vi "fits_header.vi"(0 "gfits refnum":T1, 2 "wavelength":dbl=630.2, 3 "Instru ID":string="MSSP_FeI", 4 "error in (no error)":errorcluster, 5 "start time":timestamp, 6 "total scans":dbl=190.0, 7 "end time":timestamp, 8 "Exposure":i32, 9 "num of img added":i32=1, 10 "lcvr1_2":dbl, 11 "lcvr2_4":dbl, 12 "lcvr1_4":dbl, 13 "lcvr2_2":dbl, 14 "lcvr1_1":dbl, 15 "lcvr1_3":dbl, 16 "lcvr2_1":dbl, 17 "lcvr2_3":dbl, 18 "Curr Scan":dbl, 19 "Teliscope parameters":bool) -> (20 "dup gfits refnum":T1, 27 "error out":errorcluster)   [LabVIEW 2014]
uses:
  gfitsio/gfitsio-refnum.ctl
  gfitsio/gfitsio.lvlib
  weekend/mast_controlsystem/MASTTCSGET.lvlib
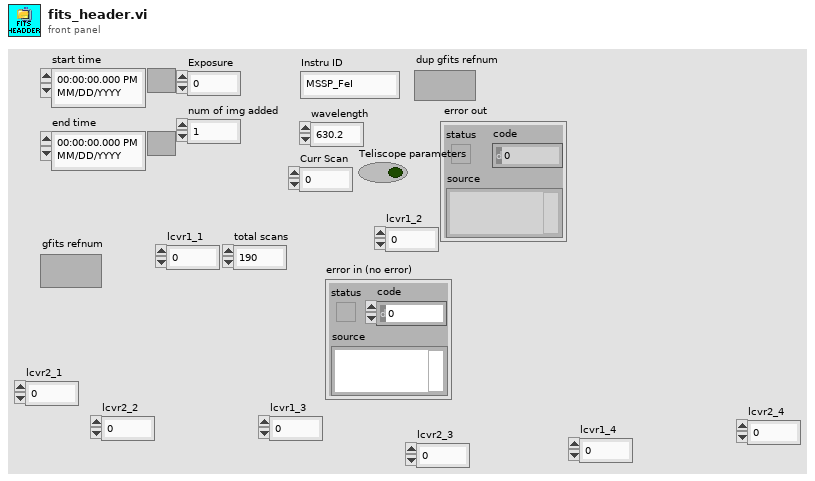
[diagram p1: front panel]
types:
  T1 = typedef "gfitsio.lvlib/gfitsio-refnum.ctl" = refnum<k1>
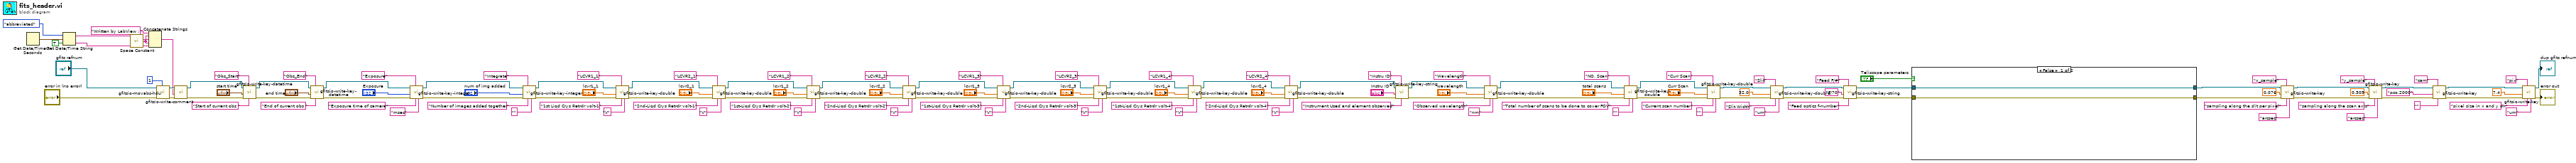
[diagram p0: block diagram]
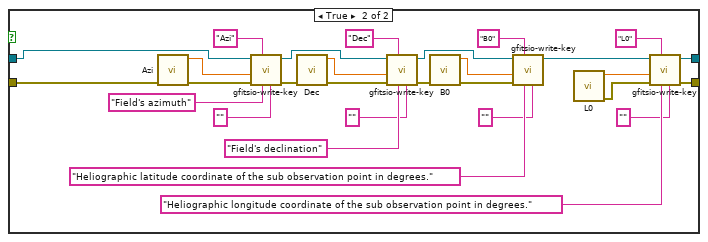
[diagram p2: hidden frame]
diagram:
  n1 = Get Date/Time In Seconds() -> (seconds since 1Jan1904=w143:timestamp)
  n2 = Get Date/Time String(date format (0)=enum16{"short", "long", "abbreviated"}."abbreviated", seconds (now)=w143, want seconds? (F)=TRUE) -> (date string=w140:string, time string=w138:string)
  n3 = call <vilib>:"Space Constant.vi"() -> ("String"=w139:string)
  n4 = Concatenate Strings("Written by LabView : " ("comment"), w139, w140, w139, w138) -> (w136:string)
  n5 = call "gfitsio-movabs-hdu.vi"("hdunum"=1, "error in (no error)"="error in (no error)", "gfits refnum"="gfits refnum") -> ("error out"=w135:errorcluster, "dup gfits refnum"=w137:T1)  [unwired: 6 in, 1 out]
  n6 = call "gfitsio-write-comment.vi"("error in (no error)"=w135, "comment"=w136, "gfits refnum"=w137) -> ("error out"=w131:errorcluster, "dup gfits refnum"=w132:T1)  [unwired: 7 in]
  n7 = call "gfitsio-write-key-datetime.vi"("comment"="Start of current obs ", "keyname"="Obs_Start", "error in (no error)"=w131, "value"="start time", "gfits refnum"=w132) -> ("error out"=w127:errorcluster, "dup gfits refnum"=w130:T1)  [unwired: 5 in]
  n8 = call "gfitsio-write-key-datetime.vi"("comment"="End of current obs ", "keyname"="Obs_End", "error in (no error)"=w127, "value"="end time", "gfits refnum"=w130) -> ("error out"=w125:errorcluster, "dup gfits refnum"=w126:T1)  [unwired: 5 in]
  n9 = call "gfitsio-write-key-integer.vi"("units"="msec", "comment"="Exposure time of camera", "keyname"="Exposure", "error in (no error)"=w125, "value"="Exposure", "gfits refnum"=w126) -> ("error out"=w114:errorcluster, "dup gfits refnum"=w118:T1)  [unwired: 4 in]
  n10 = call "gfitsio-write-key-integer.vi"("units"="", "comment"="Number of images added together", "keyname"="Integrate", "error in (no error)"=w114, "value"="num of img added", "gfits refnum"=w118) -> ("error out"=w112:errorcluster, "dup gfits refnum"=w113:T1)  [unwired: 4 in]
  n11 = call "gfitsio-write-key-double.vi"("units"="V", "comment"="1st Liqd Crys Retrdr volt-1", "keyname"="LCVR1_1", "error in (no error)"=w112, "value"="lcvr1_1", "gfits refnum"=w113) -> ("error out"=w102:errorcluster, "dup gfits refnum"=w103:T1)  [unwired: 4 in]
  n12 = call "gfitsio-write-key-double.vi"("units"="V", "comment"="2nd-Liqd Crys Retrdr volt-1", "keyname"="LCVR2_1", "error in (no error)"=w102, "value"="lcvr2_1", "gfits refnum"=w103) -> ("error out"=w96:errorcluster, "dup gfits refnum"=w97:T1)  [unwired: 4 in]
  n13 = call "gfitsio-write-key-double.vi"("units"="V", "comment"="1st-Liqd Crys Retrdr volt-2", "keyname"="LCVR1_2", "error in (no error)"=w96, "value"="lcvr1_2", "gfits refnum"=w97) -> ("error out"=w74:errorcluster, "dup gfits refnum"=w75:T1)  [unwired: 4 in]
  n14 = call "gfitsio-write-key-double.vi"("units"="V", "comment"="2nd-Liqd Crys Retrdr volt-2", "keyname"="LCVR2_2", "error in (no error)"=w74, "value"="lcvr2_2", "gfits refnum"=w75) -> ("error out"=w72:errorcluster, "dup gfits refnum"=w73:T1)  [unwired: 4 in]
  n15 = call "gfitsio-write-key-double.vi"("units"="V", "comment"="1st-Liqd Crys Retrdr volt-3", "keyname"="LCVR1_3", "error in (no error)"=w72, "value"="lcvr1_3", "gfits refnum"=w73) -> ("error out"=w70:errorcluster, "dup gfits refnum"=w71:T1)  [unwired: 4 in]
  n16 = call "gfitsio-write-key-double.vi"("units"="V", "comment"="2nd-Liqd Crys Retrdr volt-3", "keyname"="LCVR2_3", "error in (no error)"=w70, "value"="lcvr2_3", "gfits refnum"=w71) -> ("error out"=w68:errorcluster, "dup gfits refnum"=w69:T1)  [unwired: 4 in]
  n17 = call "gfitsio-write-key-double.vi"("units"="V", "comment"="1st-Liqd Crys Retrdr volt-4", "keyname"="LCVR1_4", "error in (no error)"=w68, "value"="lcvr1_4", "gfits refnum"=w69) -> ("error out"=w66:errorcluster, "dup gfits refnum"=w67:T1)  [unwired: 4 in]
  n18 = call "gfitsio-write-key-double.vi"("units"="V", "comment"="2nd-Liqd Crys Retrdr volt-4", "keyname"="LCVR2_4", "error in (no error)"=w66, "value"="lcvr2_4", "gfits refnum"=w67) -> ("error out"=w61:errorcluster, "dup gfits refnum"=w62:T1)  [unwired: 4 in]
  n19 = call "gfitsio-write-key-string.vi"("comment"="Instrument Used and element observed", "keyname"="Instru ID", "error in (no error)"=w61, "value"="Instru ID", "gfits refnum"=w62) -> ("error out"=w59:errorcluster, "dup gfits refnum"=w60:T1)  [unwired: 5 in]
  n20 = call "gfitsio-write-key-double.vi"("units"="nm", "comment"="Observed wavelength", "keyname"="Wavelength", "error in (no error)"=w59, "value"="wavelength", "gfits refnum"=w60) -> ("error out"=w51:errorcluster, "dup gfits refnum"=w54:T1)  [unwired: 4 in]
  n21 = call "gfitsio-write-key-double.vi"("units"="", "comment"="Total number of scans to be done to cover FOV", "keyname"="NO. Scan", "error in (no error)"=w51, "value"="total scans", "gfits refnum"=w54) -> ("error out"=w46:errorcluster, "dup gfits refnum"=w47:T1)  [unwired: 4 in]
  n22 = call "gfitsio-write-key-double.vi"("units"="", "comment"="Current scan number", "keyname"="Curr Scan", "error in (no error)"=w46, "value"="Curr Scan", "gfits refnum"=w47) -> ("error out"=w40:errorcluster, "dup gfits refnum"=w43:T1)  [unwired: 4 in]
  n23 = call "gfitsio-write-key-double.vi"("units"="um", "comment"="Slit Width", "keyname"="Slit", "error in (no error)"=w40, "value"=32.0, "gfits refnum"=w43) -> ("error out"=w37:errorcluster, "dup gfits refnum"=w38:T1)  [unwired: 4 in]
  n24 = call "gfitsio-write-key-string.vi"("comment"="Feed optics f-number", "keyname"="Feed F/#", "error in (no error)"=w37, "value"="F/70", "gfits refnum"=w38) -> ("error out"=w30:errorcluster, "dup gfits refnum"=w29:T1)  [unwired: 5 in]
  n25 = case shown="False" "Teliscope parameters" {
    tunnel: w30 -> [w146 w176]
    tunnel: w29 -> [w147 w173]
    tunnel: [w147 w156] -> w28
    tunnel: [w146 w155] -> w27
    frame False {
    }
    frame True {
      n26 = call "Azi.vi"("error in (no error)"=w176) -> ("error out"=w175:errorcluster, "function return"=w174:dbl)  [unwired: 9 in]
      n27 = call-poly <userlib>:"gfitsio-write-key.vi"("units"="", "comment"="Field's azimuth", "keyname"="Azi", "error in (no error)"=w175, "value"=w174, "gfits refnum"=w173) -> ("error out"=w169:errorcluster, "dup gfits refnum"=w167:T1)  [unwired: 4 in]
      n28 = call "Dec.vi"("error in (no error)"=w169) -> ("error out"=w166:errorcluster, "function return"=w168:dbl)  [unwired: 9 in]
      n29 = call-poly <userlib>:"gfitsio-write-key.vi"("units"="", "comment"="Field's declination", "keyname"="Dec", "error in (no error)"=w166, "value"=w168, "gfits refnum"=w167) -> ("error out"=w162:errorcluster, "dup gfits refnum"=w154:T1)  [unwired: 4 in]
      n30 = call "B0.vi"("error in (no error)"=w162) -> ("error out"=w153:errorcluster, "function return"=w152:dbl)  [unwired: 9 in]
      n31 = call-poly <userlib>:"gfitsio-write-key.vi"("units"="", "comment"="Heliographic latitude coordinate of the sub observation point in degrees.", "keyname"="B0", "error in (no error)"=w153, "value"=w152, "gfits refnum"=w154) -> ("dup gfits refnum"=w148:T1)  [unwired: 4 in, 1 out]
      n32 = call "L0.vi"() -> ("error out"=w160:errorcluster, "function return"=w161:dbl)  [unwired: 10 in]
      n33 = call-poly <userlib>:"gfitsio-write-key.vi"("units"="", "comment"="Heliographic longitude coordinate of the sub observation point in degrees.", "keyname"="L0", "error in (no error)"=w160, "value"=w161, "gfits refnum"=w148) -> ("error out"=w155:errorcluster, "dup gfits refnum"=w156:T1)  [unwired: 4 in]
    }
  }
  n34 = call-poly <userlib>:"gfitsio-write-key.vi"("units"="arcsec", "comment"="sampling along the slit per pixel", "keyname"="x_sample", "error in (no error)"=w27, "value"=0.076, "gfits refnum"=w28) -> ("error out"=w22:errorcluster, "dup gfits refnum"=w23:T1)  [unwired: 4 in]
  n35 = call-poly <userlib>:"gfitsio-write-key.vi"("units"="arcsec", "comment"="sampling along the scan axis", "keyname"="y_sample", "error in (no error)"=w22, "value"=0.309, "gfits refnum"=w23) -> ("error out"=w14:errorcluster, "dup gfits refnum"=w16:T1)  [unwired: 4 in]
  n36 = call-poly <userlib>:"gfitsio-write-key.vi"("comment"="", "keyname"="cam", "error in (no error)"=w14, "value"="pco.2000", "gfits refnum"=w16) -> ("error out"=w4:errorcluster, "dup gfits refnum"=w11:T1)  [unwired: 5 in]
  n37 = call-poly <userlib>:"gfitsio-write-key.vi"("units"="um", "comment"="pixel size in x and y dir", "keyname"="pix", "error in (no error)"=w4, "value"=7.4, "gfits refnum"=w11) -> ("error out"=→"error out":errorcluster, "dup gfits refnum"=→"dup gfits refnum":T1)  [unwired: 4 in]
